vi "Compare_Calib_Files.vi"(0 "Calib file New":path=path "/iMac_3 HD/Users/Hong(6%)/calib/XW Ch 1 7_10_02_6", 1 "Calib file Orig":path=path "/iMac_3 HD/Users/Hong(6%)/calib/XW Ch 1 7_10_02_5", 2 "Instrument type":T1=enum."Cross wire velocity") -> (3 "Calib name":string, 4 "% Change":dbl format="%.2f", 5 "Calib Time Separation (Hours)":dbl format="%.2f", 6 "Temperature Change":dbl)   [LabVIEW 2022 SP3]
uses:
  Controls/Cal_Inst_type.ctl
  Controls/Inst_type.ctl
  <vilib>/Analysis/baseanly.llb/Mean (DBL).vi
  <vilib>/Analysis/NI_AALBase.lvlib
panel:
  out "U1 % Change":dbl format="%.4f"
  out "U2 % Change":dbl format="%.4f"
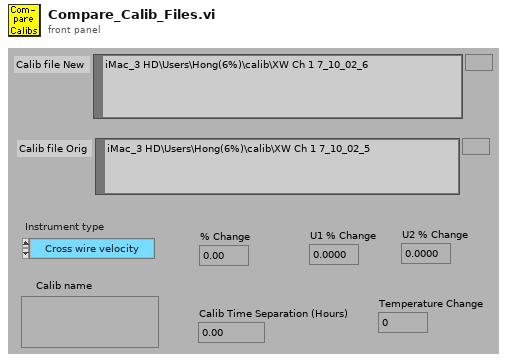
[diagram p1: front panel]
types:
  T1 = typedef "Cal_Inst_type.ctl" = enum16{"Propeller anemometer", "Pressure Transducer", "Hot wire", "Cross wire velocity", "Cross wire angle", "Generic Linear", "Generic Polynomial", "Poly Fit Special", "Fast FID", "Thermocouple", "Cold wire", "Pulsed Wire"}
  T2 = typedef "Inst_type.ctl" = enum16{"Raw voltage", "Raw with zero offsetting", "Propeller anemometer", "Pressure Transducer", "Pitot-static tube", "Hot wire", "Cross wire 1", "Cross wire 2", "Generic Linear", "Generic Polynomial", "Generic BackPoly", "Fast FID", "Thermocouple", "Cold wire", "Pulsed Wire", "LDA Vel", "LDA Tran time", "LDA Arr time", "Microphone"}
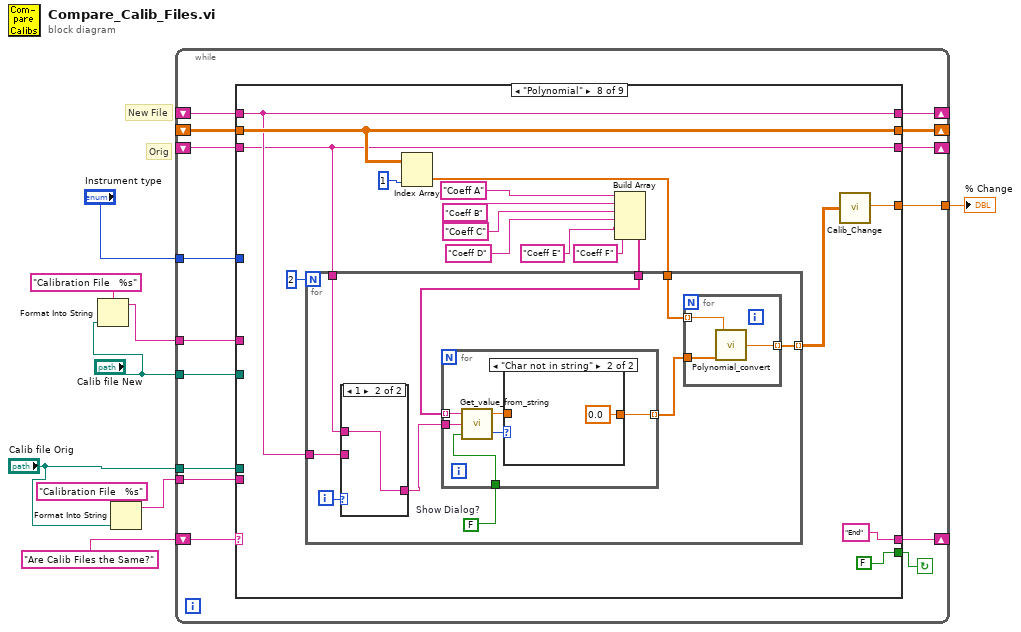
[diagram p0: block diagram]
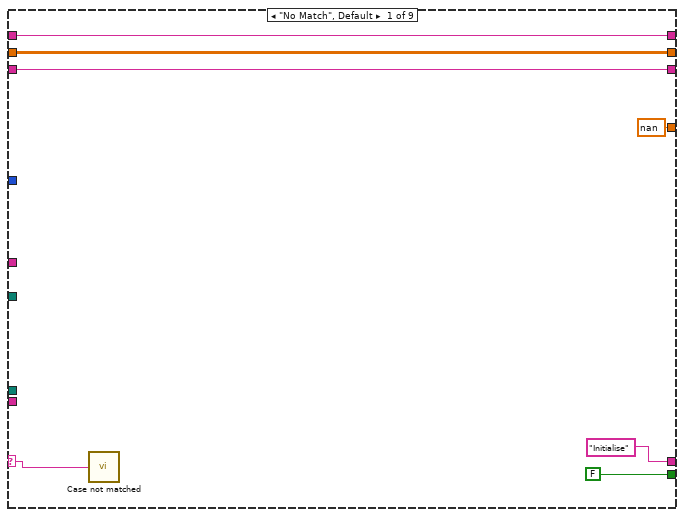
[diagram p2: hidden frame]
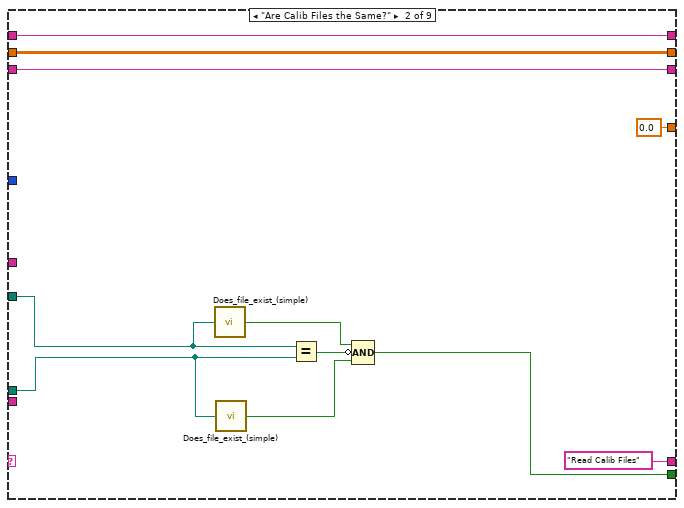
[diagram p3: hidden frame]
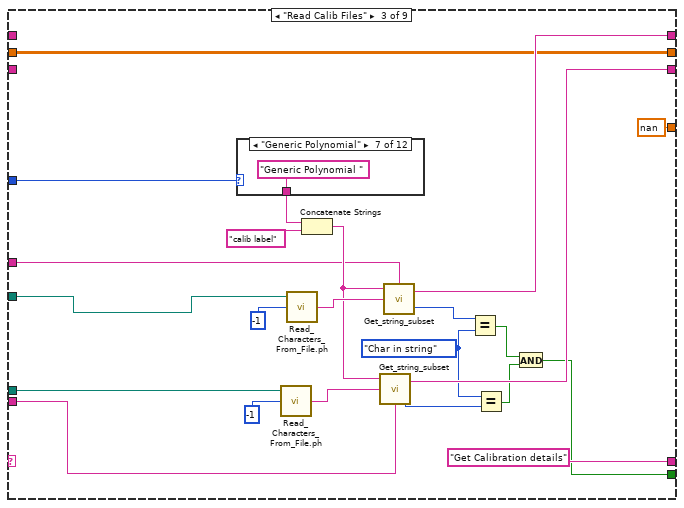
[diagram p4: hidden frame]
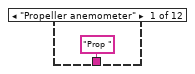
[diagram p5: hidden frame]
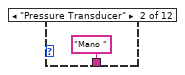
[diagram p6: hidden frame]
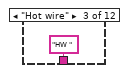
[diagram p7: hidden frame]
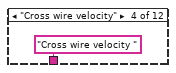
[diagram p8: hidden frame]
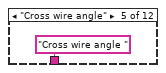
[diagram p9: hidden frame]
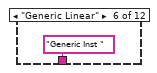
[diagram p10: hidden frame]
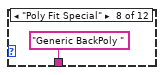
[diagram p11: hidden frame]
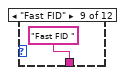
[diagram p12: hidden frame]
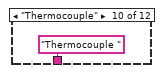
[diagram p13: hidden frame]
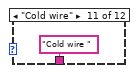
[diagram p14: hidden frame]
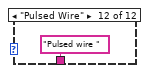
[diagram p15: hidden frame]
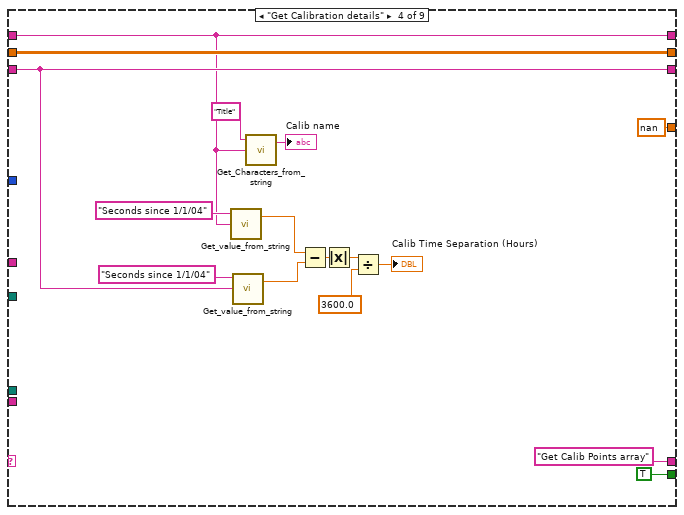
[diagram p16: hidden frame]
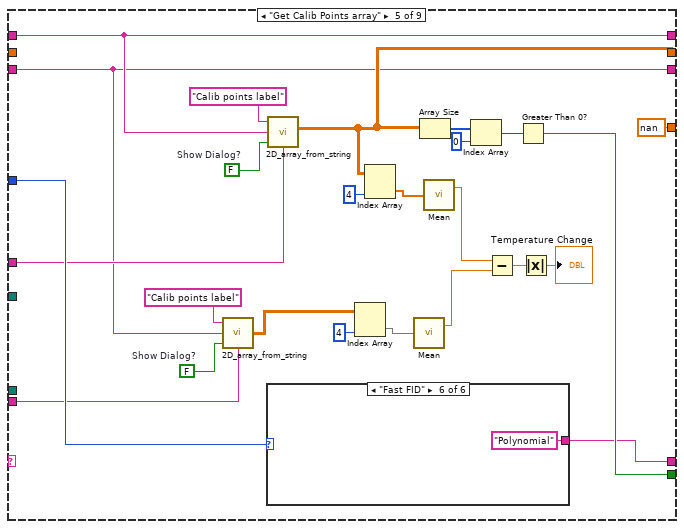
[diagram p17: hidden frame]
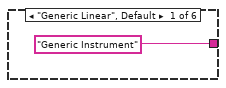
[diagram p18: hidden frame]
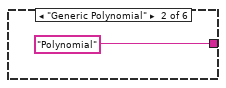
[diagram p19: hidden frame]
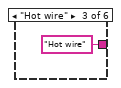
[diagram p20: hidden frame]
diagram:
  # "New File"
  # "Orig"
  n1 = Format Into String(format string="Calibration File   %s", "Calib file New") -> (resulting string=w2:string)  [unwired: 2 in, 1 out]
  n2 = Format Into String(format string="Calibration File   %s", "Calib file Orig") -> (resulting string=w1:string)  [unwired: 2 in, 1 out]
  n3 = while {
    tunnel: "Calib file Orig" -> [w12]
    tunnel: "Calib file New" -> [w13]
    tunnel: [w14] -> w7
    shift-left: _ -> [w15]
    shift-right: [w16] -> _
    shift-left: _ -> [w17]
    shift-right: [w19] -> _
    tunnel: "Instrument type" -> [w21]
    shift-left: _ -> [w18]
    shift-right: [w20] -> _
    shift-left: "Are Calib Files the Same?" -> [w22]
    shift-right: [w23] -> _
    tunnel: w2 -> [w11]
    tunnel: w1 -> [w10]
    stop <- w24 continue-if-true
    n4 = case shown="\"Polynomial\"" w22 {
      selector: w22 -> [w25 _ _ _ _ _ _ _ _]
      tunnel: [FALSE w34 w48 TRUE w111 FALSE FALSE FALSE FALSE] -> w24
      tunnel: ["Initialise" "Read Calib Files" "Get Calibration details" "Get Calib Points array" w109 "End" "End" "End" "End"] -> w23
      tunnel: w21 -> [_ _ w60 _ w115 _ _ _ _]
      tunnel: [w29 w42 w59 w79 w116 w143 w152 w182 w238] -> w20
      tunnel: [w28 w40 w56 w90 w102 w136 w151 w181 w232] -> w19
      tunnel: w18 -> [w29 w42 _ w79 w116 w143 w152 w182 w238]
      tunnel: w17 -> [w28 w40 _ w90 w102 w136 w151 w181 w232]
      tunnel: [w27 w41 w55 w93 w107 w150 w160 w195 w248] -> w16
      tunnel: w15 -> [w27 w41 w55 w93 _ w150 w160 w195 w248]
      tunnel: [nan ("% Change") 0.0 ("% Change") nan ("% Change") nan ("% Change") nan ("% Change") w148 w155 w190 w244] -> w14
      tunnel: w13 -> [_ w33 w45 _ _ _ _ _ _]
      tunnel: w12 -> [_ w32 w46 _ _ _ _ _ _]
      tunnel: w11 -> [_ _ w44 _ w108 w126 _ _ w219]
      tunnel: w10 -> [_ _ w43 _ w101 w125 _ _ w218]
      frame "No Match", Default {
        n5 = call "Case not matched.vi"("Case Name not Matched"=w25) -> ()
      }
      frame "Are Calib Files the Same?" {
        n6 = call "Does_file_exist_(simple).vi"("Pathname"=w33) -> ("exists?"=w37:bool)
        n7 = call "Does_file_exist_(simple).vi"("Pathname"=w32) -> ("exists?"=w35:bool)
        n8 = Equal?(x=w33, y=w32) -> (x = y?=w36:bool)
        n9 = Compound Arithmetic op=AND(w37, invert w36, w35) -> (w34:bool)
      }
      frame "Read Calib Files" {
        w52 = enum16{"Char in string", "Char not in string"}."Char in string" ("Status")
        n10 = case shown="\"Generic Polynomial\"" w60 {
          tunnel: ["Prop " "Mano " "HW " "Cross wire velocity " "Cross wire angle " "Generic Inst " "Generic Polynomial " "Generic BackPoly " "Fast FID " "Thermocouple " "Cold wire " "Pulsed wire "] -> w61
          frame "Propeller anemometer" {
          }
          frame "Pressure Transducer" {
          }
          frame "Hot wire" {
          }
          frame "Cross wire velocity" {
          }
          frame "Cross wire angle" {
          }
          frame "Generic Linear" {
          }
          frame "Generic Polynomial" {
          }
          frame "Poly Fit Special" {
          }
          frame "Fast FID" {
          }
          frame "Thermocouple" {
          }
          frame "Cold wire" {
          }
          frame "Pulsed Wire" {
          }
        }
        n11 = call "Read_Characters_From_File.ph.vi"("file path (dialog if empty)"=w46, "number of characters (all:-1)"=-1) -> ("character string"=w58:string)  [unwired: 7 out]
        n12 = call "Read_Characters_From_File.ph.vi"("file path (dialog if empty)"=w45, "number of characters (all:-1)"=-1) -> ("character string"=w63:string)  [unwired: 7 out]
        n13 = Concatenate Strings(w61, "calib label") -> (w54:string)
        n14 = call "Get_string_subset.vi"("String Name"=w43, "String to split"=w58, "File Label"=w54) -> ("Status"=w51:enum16{"Char in string", "Char not in string"}, "Output string"=w56:string)  [unwired: 1 in]
        n15 = call "Get_string_subset.vi"("String Name"=w44, "String to split"=w63, "File Label"=w54) -> ("Status"=w53:enum16{"Char in string", "Char not in string"}, "Output string"=w59:string)  [unwired: 1 in]
        n16 = Equal?(x=w53, y=w52) -> (x = y?=w49:bool)
        n17 = Equal?(x=w52, y=w51) -> (x = y?=w50:bool)
        n18 = And(x=w49, y=w50) -> (x .and. y?=w48:bool)
      }
      frame "Get Calibration details" {
        n19 = call "Get_value_from_string.vi"("Input string"=w79, "Variable name"="Seconds since 1/1/04") -> ("Value"=w89:dbl)  [unwired: 1 in, 1 out]
        n20 = call "Get_value_from_string.vi"("Input string"=w90, "Variable name"="Seconds since 1/1/04") -> ("Value"=w88:dbl)  [unwired: 1 in, 1 out]
        n21 = call "Get_Characters_from_string.vi"("Input string"=w79, "Variable name"="Title") -> ("Value"=→"Calib name":string)  [unwired: 1 in, 1 out]
        n22 = Subtract(x=w89, y=w88) -> (x-y=w87:dbl)
        n23 = Absolute Value(x=w87) -> (abs(x)=w78:dbl)
        n24 = Divide(x=w78, y=3600.0) -> (x/y=→"Calib Time Separation (Hours)":dbl)
      }
      frame "Get Calib Points array" {
        w103 = FALSE  # Show Dialog?
        w118 = FALSE  # Show Dialog?
        n25 = call "2D_array_from_string.vi"("String Name"=w101, "Show Dialog?"=w103, "Input string"=w102, "Array title"="Calib points label") -> ("2D data array"=w98:dbl[][])
        n26 = case shown="\"Fast FID\"" w115 {
          tunnel: ["Generic Instrument" "Polynomial" "Hot wire" "Cross wire velocity" "Polynomial" "Polynomial"] -> w109
          frame "Generic Linear", Default {
          }
          frame "Generic Polynomial" {
          }
          frame "Hot wire" {
          }
          frame "Cross wire velocity" {
          }
          frame "Cold wire" {
          }
          frame "Fast FID" {
          }
        }
        n27 = call "2D_array_from_string.vi"("String Name"=w108, "Show Dialog?"=w118, "Input string"=w116, "Array title"="Calib points label") -> ("2D data array"=w107:dbl[][])
        n28 = Index Array(array=w98, index (col)=4 ("disabled index (col)")) -> (element=w100:dbl[])  [unwired: 1 in]
        n29 = Index Array(array=w107, index (col)=4 ("disabled index (col)")) -> (element=w105:dbl[])  [unwired: 1 in]
        n30 = call-poly <vilib>:"Mean.vi"("X"=w100) -> ("mean"=w96:dbl)  [unwired: 1 out]
        n31 = Array Size(array=w107) -> (size(s)=w114:i32[])
        n32 = call-poly <vilib>:"Mean.vi"("X"=w105) -> ("mean"=w97:dbl)  [unwired: 1 out]
        n33 = Index Array(array=w114, index=0 ("Index")) -> (element=w112:i32)
        n34 = Subtract(x=w97, y=w96) -> (x-y=w95:dbl)
        n35 = Greater Than 0?(x=w112) -> (x > 0?=w111:bool)
        n36 = Absolute Value(x=w95) -> (abs(x)=→"Temperature Change":dbl)
      }
      frame "Hot wire" {
        w140 = TRUE  # Take New Data?
        w139 = FALSE  # Show Dialog?
        w141 = TRUE  # Take New Data?
        w142 = FALSE  # Show Dialog?
        # "New Calib"
        # "Original calib corrected to new calib temperture"
        n37 = call "Get_Coeff_Fr_String.vi"("String Name"=w126, "Take New Data?"=w141, "Prefix"="", "Show Dialog?"=w142, "Sub String"=w143, "Inst type"=Inst_type."Hot wire") -> ("Calib Constants"=w133:dbl[])  [unwired: 3 in, 1 out]
        n38 = call "Get_Coeff_Fr_String.vi"("String Name"=w125, "Take New Data?"=w140, "Prefix"="", "Show Dialog?"=w139, "Sub String"=w136, "Inst type"=Inst_type."Hot wire") -> ("Calib Constants"=w129:dbl[])  [unwired: 3 in, 1 out]
        n39 = Index Array(array=w133, index=3) -> (element=w128:dbl)
        n40 = Index Array(array=w150, index (col)=1 ("Index")) -> (element=w135:dbl[])  [unwired: 1 in]
        n41 = call "HW_Linearise_+_temp_comp.vi"("Caib const"=w133, "HW voltage"=w135) -> ("Velocity"=w132:dbl[])  [unwired: 4 in, 1 out]
        n42 = call "SW_Type_1a_correction.vi"("Tmeas (degC)"=w128, "Calib consts."=w129) -> ("Corrected calib consts."=w127:dbl[])
        n43 = call "HW_Linearise_+_temp_comp.vi"("Caib const"=w127, "HW voltage"=w135) -> ("Velocity"=w131:dbl[])  [unwired: 4 in, 1 out]
        n44 = Build Array(w132, w131) -> (w130:dbl[][])
        n45 = call "Calib_Change.vi"("Eng Units"=w130) -> ("% Change"=w148:dbl)
      }
      frame "Generic Instrument" {
        n46 = Index Array(array=w160, index (col)=1 ("Index")) -> (element=w157:dbl[])  [unwired: 1 in]
        n47 = for {
          N: 2 -> [_]
          tunnel: w151 -> [w170]
          tunnel: w152 -> [w166]
          tunnel: w157 -> [w163]
          tunnel: [w161] -> w156 mode=indexing
          i -> [w171]
          w167 = FALSE  # Show Dialog?
          n48 = case shown="1" w171 {
            tunnel: w170 -> [_ w178]
            tunnel: [w177 w178] -> w169
            tunnel: w166 -> [w177 _]
            frame 0, Default {
            }
            frame 1 {
            }
          }
          n49 = call "Get_value_from_string.vi"("Show Dialog?"=w167, "Input string"=w169, "Variable name"="Coeff A") -> ("Value"=w168:dbl)  [unwired: 1 out]
          n50 = call "Get_value_from_string.vi"("Show Dialog?"=w167, "Input string"=w169, "Variable name"="Coeff B") -> ("Value"=w162:dbl)  [unwired: 1 out]
          n51 = for {
            tunnel: w168 -> [w175]
            tunnel: w163 -> [w174] mode=indexing
            tunnel: w162 -> [w173]
            tunnel: [w172] -> w161 mode=indexing
            n52 = Subtract(x=w174, y=w175) -> (x-y=w176:dbl)
            n53 = Divide(x=w176, y=w173) -> (x/y=w172:dbl)
          }
        }
        n54 = call "Calib_Change.vi"("Eng Units"=w156) -> ("% Change"=w155:dbl)
      }
      frame "Polynomial" {
        n55 = Index Array(array=w195, index (col)=1 ("Index")) -> (element=w192:dbl[])  [unwired: 1 in]
        n56 = Build Array("Coeff A", "Coeff B", "Coeff C", "Coeff D", "Coeff E", "Coeff F") -> (w185:string[])
        n57 = for {
          N: 2 -> [_]
          tunnel: w181 -> [w203]
          tunnel: w182 -> [w202]
          tunnel: w192 -> [w201]
          tunnel: [w200] -> w191 mode=indexing
          tunnel: w185 -> [w197]
          i -> [w204]
          w199 = FALSE  # Show Dialog?
          n58 = case shown="1" w204 {
            tunnel: w203 -> [_ w217]
            tunnel: [w216 w217] -> w198
            tunnel: w202 -> [w216 _]
            frame 0, Default {
            }
            frame 1 {
            }
          }
          n59 = for {
            tunnel: w199 -> [w209]
            tunnel: w198 -> [w208]
            tunnel: w197 -> [w207] mode=indexing
            tunnel: [w205] -> w196 mode=indexing
            n60 = call "Get_value_from_string.vi"("Show Dialog?"=w209, "Input string"=w208, "Variable name"=w207) -> ("Status"=w210:enum16{"Char in string", "Char not in string"}, "Value"=w206:dbl)
            n61 = case shown="\"Char not in string\"" w210 {
              tunnel: w206 -> [w211 _]
              tunnel: [w211 0.0 ("Value")] -> w205
              frame "Char in string" {
              }
              frame "Char not in string" {
              }
            }
          }
          n62 = for {
            tunnel: w201 -> [w215] mode=indexing
            tunnel: [w214] -> w200 mode=indexing
            tunnel: w196 -> [w213]
            n63 = call "Polynomial_convert.vi"("Calib constants"=w213, "Voltage"=w215) -> ("Eng Values"=w214:dbl)  [unwired: 4 out]
          }
        }
        n64 = call "Calib_Change.vi"("Eng Units"=w191) -> ("% Change"=w190:dbl)
      }
      frame "Cross wire velocity" {
        w235 = TRUE  # Take New Data?
        w234 = FALSE  # Show Dialog?
        w239 = TRUE  # Take New Data?
        w240 = FALSE  # Show Dialog?
        w223 = Inst_type."Cross wire 1" ("Inst type")
        # "U2"
        # "U1"
        n65 = Index Array(array=w248, index (col)=1 ("Index")) -> (element=w231:dbl[])  [unwired: 1 in]
        n66 = Index Array(array=w248, index (col)=2 ("Index")) -> (element=w230:dbl[])  [unwired: 1 in]
        n67 = call "Get_Coeff_Fr_String.vi"("String Name"=w219, "Take New Data?"=w239, "Prefix"="", "Show Dialog?"=w240, "Sub String"=w238, "Inst type"=w223) -> ("Calib Constants"=w236:dbl[])  [unwired: 3 in, 1 out]
        n68 = call "Get_Coeff_Fr_String.vi"("String Name"=w218, "Take New Data?"=w235, "Prefix"="", "Show Dialog?"=w234, "Sub String"=w232, "Inst type"=w223) -> ("Calib Constants"=w221:dbl[])  [unwired: 3 in, 1 out]
        n69 = Index Array(array=w236, index=9) -> (element=w222:dbl)
        n70 = call "XW_Type_1a_correction.vi"("Tmeas (degC)"=w222, "Calib consts."=w221) -> ("Corrected calib consts."=w220:dbl[])
        n71 = call "XW_Linearise_+_temp_comp.vi"("XW2 voltage"=w230, "Calib const"=w236, "XW1 voltage"=w231) -> ("U2"=w225:dbl[], "U1"=w226:dbl[])  [unwired: 5 in, 2 out]
        n72 = call "XW_Linearise_+_temp_comp.vi"("XW2 voltage"=w230, "Calib const"=w220, "XW1 voltage"=w231) -> ("U2"=w227:dbl[], "U1"=w229:dbl[])  [unwired: 5 in, 2 out]
        n73 = Build Array(w226, w229) -> (w228:dbl[][])
        n74 = Build Array(w225, w227) -> (w224:dbl[][])
        n75 = call "Calib_Change.vi"("Eng Units"=w228) -> ("% Change"=w246:dbl)
        "U1 % Change" <- w246
        n76 = call "Calib_Change.vi"("Eng Units"=w224) -> ("% Change"=w245:dbl)
        "U2 % Change" <- w245
        n77 = Greater?(x=w246, y=w245) -> (0:w247:bool)
        n78 = Select(t=w246, s=w247, f=w245) -> (s? t:f=w244:dbl)
      }
    }
  }
  "% Change" <- w7
